vi "modulation.vi"() -> ()   [LabVIEW 2017]
uses:
  <vilib>/measure/NI_MABase.lvlib
panel:
  in  "stop":bool
  out "modulated signal":waveform(dbl)[](graph)
  out "main signal":waveform(dbl)[](graph)
  out "carrier":waveform(dbl)(graph)
  in  "path 3":path
  in  "modulation index":dbl(knob) scale=0.0..3.0
  in  "carrier":dbl(knob) scale=0.0..1000.0
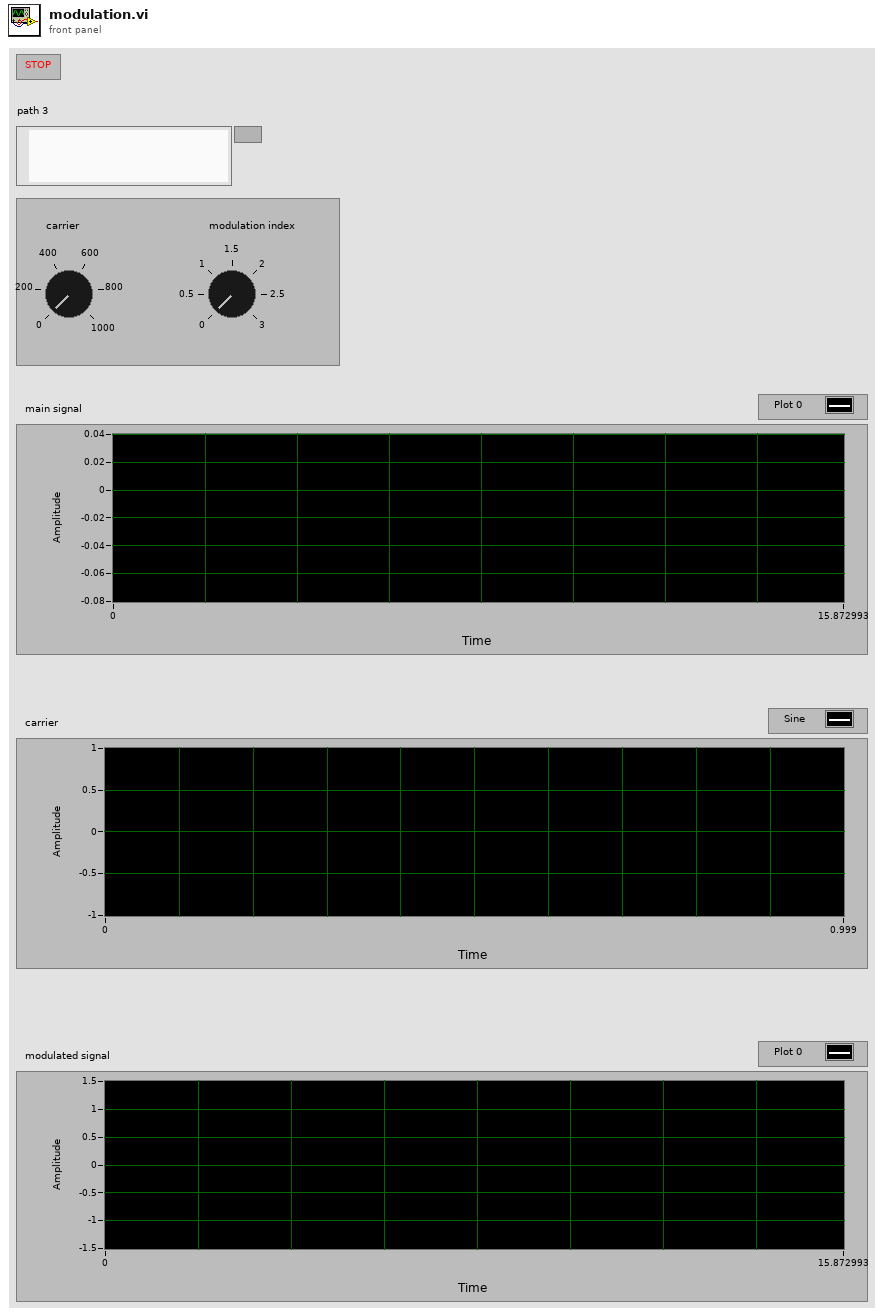
[diagram p1: front panel]
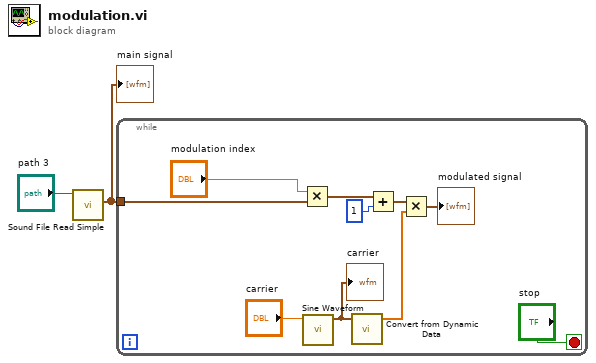
[diagram p0: block diagram]
diagram:
  n1 = call <vilib>:"Sound File Read Simple.vi"("path"="path 3") -> ("data"=w1:waveform(dbl)[])  [unwired: 7 in, 3 out]
  "main signal" <- w1
  n2 = while {
    tunnel: w1 -> [w11]
    stop <- "stop" stop-if-true
    n3 = Multiply(x="modulation index", y=w11) -> (x*y=w12:waveform(dbl)[])
    n4 = call <vilib>:"Sine Waveform.vi"("frequency"="carrier") -> ("signal out"=w4:waveform(dbl))  [unwired: 9 in, 1 out]
    "carrier" <- w4
    n5 = call "Convert from Dynamic Data"("Dynamic Data Type"=w4) -> ("Array"=w7:dbl[])  [unwired: 3 in]
    n6 = Add(x=w12, y=1) -> (x+y=w9:waveform(dbl)[])
    n7 = Multiply(x=w9, y=w7) -> (x*y=→"modulated signal":waveform(dbl)[])
  }
